vi "acqTest.vi"() -> ()   [LabVIEW 2019]
uses:
  <vilib>/Utility/Variable/NI_VariableUtilities.lvlib
panel:
  in  "Acq State":bool
  in  "stop":bool
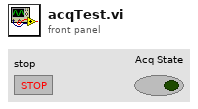
[diagram p1: front panel]
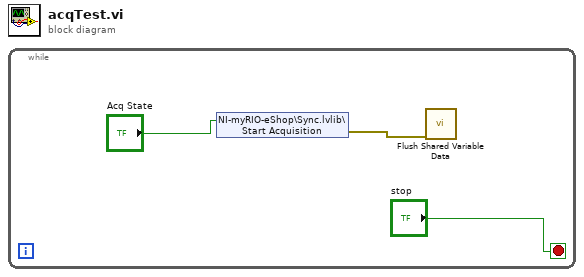
[diagram p0: block diagram]
diagram:
  n1 = while {
    stop <- "stop" stop-if-true
    n2 = shared-variable "NI-myRIO-eShop\\Sync.lvlib\\Start Acquisition"("Acq State") -> (error out=w3:errorcluster)  [unwired: 1 in]
    n3 = call <vilib>:"Flush Shared Variable Data.vi"("error in (no error)"=w3) -> ()  [unwired: 10 in, 1 out]
  }
